vi "MegaAnalysis5.vi"() -> ()   [LabVIEW 2016] (continued)
                          n1538 = Multiply(x=w3837, y=6.283185307179586) -> (x*y=w3835:ext[])
                          n1539 = Divide(x=w3831, y=w3826) -> (x/y=w3839:ext[])
                          n1540 = Add(x=w3835, y=w3829) -> (x+y=w3832:ext[])
                          n1541 = Negate(x=w3839) -> (-x=w3838:ext[])
                          n1542 = Cosine(x=w3832) -> (cos(x)=w3833:ext[])
                          n1543 = Exponential(1:w3838) -> (0:w3834:ext[])
                          n1544 = Compound Arithmetic op=MULTIPLY(w3828, w3834, w3833) -> (w3825:ext[])
                          n1545 = call "writebinary.vi"(7:w3821, "base path"=w3823, "file index"=w3824, "data column"="dati", "data"=w3825) -> ()  [unwired: 7 out]
                        }
                        frame 2 {
                          w3843 = "dati"
                          n1546 = call "readbinary.vi"(7:w3840, "base path"=w3841, "file index"=w3842, "data column"="bcli") -> ("data"=w3846:ext[])  [unwired: 7 out]
                          n1547 = Divide(x=w3850, y=w3846) -> (x/y=w3858:ext[])
                          n1548 = Multiply(x=w3858, y=6.283185307179586) -> (x*y=w3856:ext[])
                          n1549 = call "readbinary.vi"(7:w3840, "base path"=w3841, "file index"=w3842, "data column"=w3843) -> ("data"=w3847:ext[])  [unwired: 7 out]
                          n1550 = Divide(x=w3851, y=w3846) -> (x/y=w3860:ext[])
                          n1551 = Add(x=w3856, y=w3849) -> (x+y=w3853:ext[])
                          n1552 = Negate(x=w3860) -> (-x=w3859:ext[])
                          n1553 = Cosine(x=w3853) -> (cos(x)=w3854:ext[])
                          n1554 = Exponential(1:w3859) -> (0:w3855:ext[])
                          n1555 = Compound Arithmetic op=MULTIPLY(w3848, w3855, w3854) -> (w3852:ext[])
                          n1556 = Subtract(x=w3847, y=w3852) -> (x-y=w3844:ext[])
                          n1557 = call "writebinary.vi"(7:w3840, "base path"=w3841, "file index"=w3842, "data column"=w3843, "data"=w3844) -> ()  [unwired: 7 out]
                        }
                        frame 3 {
                          w3864 = "dati"
                          n1558 = call "readbinary.vi"(7:w3861, "base path"=w3862, "file index"=w3863, "data column"="bcli") -> ("data"=w3866:ext[])  [unwired: 7 out]
                          n1559 = Reciprocal(x=w3866) -> (1/x=w3873:ext[])
                          n1560 = call "readbinary.vi"(7:w3861, "base path"=w3862, "file index"=w3863, "data column"=w3864) -> ("data"=w3867:ext[])  [unwired: 7 out]
                          n1561 = Index Array(array=w3873, index=2) -> (element=w3882:ext)
                          n1562 = Index Array(array=w3873, index=1) -> (element=w3883:ext)
                          n1563 = call <vilib>:"General Polynomial Fit.vi"("Y"=w3867, "polynomial order"="poly sub", "X"=w3873) -> ("Best Polynomial Fit"=w3871:dbl[])  [unwired: 9 in, 3 out]
                          n1564 = Subtract(x=w3883, y=w3882) -> (x-y=w3881:ext)
                          n1565 = Absolute Value(x=w3881) -> (abs(x)=w3880:ext)
                          n1566 = Reciprocal(x=w3880) -> (1/x=w3879:ext)
                          "sampling freq" <- w3879
                          n1567 = Subtract(x=w3867, y=w3871) -> (x-y=w3872:ext[])
                          n1568 = call-poly <vilib>:"Butterworth Filter.vi"("order"="order", "filter type"="filter type", "low cutoff freq: fl"="low cutoff", "high cutoff freq: fh"="high cutoff", "sampling freq: fs"=w3879, "X"=w3872) -> ("Filtered X"=w3869:dbl[])  [unwired: 1 in, 2 out]
                          n1569 = Add(x=w3869, y=w3871) -> (x+y=w3868:dbl[])
                          n1570 = case shown="False" "?" {
                            tunnel: w3869 -> [w3888 _]
                            tunnel: w3868 -> [_ w3895]
                            tunnel: w3864 -> [_ w3894]
                            tunnel: w3863 -> [w3889 w3893]
                            tunnel: w3862 -> [w3890 w3892]
                            tunnel: w3861 -> [w3886 w3891]
                            frame False {
                              n1571 = call "writebinary.vi"(7:w3886, "base path"=w3890, "file index"=w3889, "data column"="temp", "data"=w3888) -> ()  [unwired: 7 out]
                            }
                            frame True {
                              n1572 = call "writebinary.vi"(7:w3891, "base path"=w3892, "file index"=w3893, "data column"=w3894, "data"=w3895) -> ()  [unwired: 7 out]
                            }
                          }
                        }
                        frame 4 {
                          n1573 = call "readbinary.vi"(7:w3896, "base path"=w3898, "file index"=w3899, "data column"="timi") -> ("data"=w3903:ext[])  [unwired: 7 out]
                          n1574 = Multiply(x=w3903, y=6.283185307179586) -> (x*y=w3916:ext[])
                          n1575 = Multiply(x=w3916, y="f") -> (x*y=w3914:ext[])
                          n1576 = Add(x=w3914, y="phase") -> (x+y=w3912:ext[])
                          n1577 = call "readbinary.vi"(7:w3896, "base path"=w3898, "file index"=w3899, "data column"="bcli") -> ("data"=w3897:ext[])  [unwired: 7 out]
                          n1578 = Cosine(x=w3912) -> (cos(x)=w3911:ext[])
                          n1579 = Multiply(x=w3911, y="amp") -> (x*y=w3905:ext[])
                          n1580 = Divide(x="gamma", y=w3897) -> (x/y=w3908:ext[])
                          n1581 = Negate(x=w3908) -> (-x=w3907:ext[])
                          n1582 = Exponential(1:w3907) -> (0:w3906:ext[])
                          n1583 = Multiply(x=w3905, y=w3906) -> (x*y=w3901:ext[])
                          n1584 = call "writebinary.vi"(7:w3896, "base path"=w3898, "file index"=w3899, "data column"="dati", "data"=w3901) -> ()  [unwired: 7 out]
                        }
                      }
                    }
                  }
                  frame #5 {
                    n1585 = for {
                      tunnel: w3925 -> [_] mode=indexing
                      tunnel: "subtraction type" -> [w3935]
                      tunnel: "algorithm" -> [w3934]
                      tunnel: "polynomial order" -> [w3933]
                      tunnel: w3921 -> [w3928]
                      tunnel: "background subtraction method" -> [w3931]
                      tunnel: w3919 -> [w3927]
                      tunnel: [w3926] -> w3918 mode=indexing
                      i -> [w3929]
                      w3930 = "dati"
                      n1586 = call "readbinary.vi"(7:w3927, "base path"=w3928, "file index"=w3929, "data column"=w3930) -> ("data"=w3932:ext[])  [unwired: 7 out]
                      n1587 = case shown="2" w3935 {
                        tunnel: w3932 -> [w3952 w3962 w3973 w3980]
                        tunnel: [w3951 w3963 w3970 w3983] -> w3926
                        tunnel: w3934 -> [_ w3960 w3968 w3979]
                        tunnel: w3933 -> [_ w3959 w3969 w3978]
                        tunnel: w3929 -> [_ w3956 _ _]
                        tunnel: w3928 -> [_ w3955 _ _]
                        tunnel: w3927 -> [_ w3954 _ _]
                        frame 0, Default {
                          n1588 = Multiply(x=w3952, y=0) -> (x*y=w3951:ext[])
                        }
                        frame 1 {
                          n1589 = call "readbinary.vi"(7:w3954, "base path"=w3955, "file index"=w3956, "data column"="temp") -> ("data"=w3958:ext[])  [unwired: 7 out]
                          n1590 = Subtract(x=w3962, y=w3958) -> (x-y=w3961:ext[])
                          n1591 = Array Size(array=w3962) -> (size(s)=w3965:i32)
                          n1592 = for {
                            N: w3965 -> [_]
                            tunnel: [w3967] -> w3966 mode=indexing
                            i -> [w3967]
                          }
                          n1593 = Divide(x=w3966, y=w3965) -> (x/y=w3964:dbl[])
                          n1594 = call <vilib>:"General Polynomial Fit.vi"("Y"=w3961, "polynomial order"=w3959, "X"=w3964, "algorithm"=w3960) -> ("Best Polynomial Fit"=w3963:dbl[])  [unwired: 8 in, 3 out]
                        }
                        frame 2 {
                          n1595 = Natural Logarithm(1:w3973) -> (0:w3971:ext[])
                          n1596 = Array Size(array=w3973) -> (size(s)=w3975:i32)
                          n1597 = for {
                            N: w3975 -> [_]
                            tunnel: [w3977] -> w3976 mode=indexing
                            i -> [w3977]
                          }
                          n1598 = Divide(x=w3976, y=w3975) -> (x/y=w3974:dbl[])
                          n1599 = call <vilib>:"General Polynomial Fit.vi"("Y"=w3971, "polynomial order"=w3969, "X"=w3974, "algorithm"=w3968) -> ("Best Polynomial Fit"=w3972:dbl[])  [unwired: 8 in, 3 out]
                          n1600 = Exponential (Arg) -1(1:w3972) -> (0:w3970:dbl[])
                        }
                        frame 3 {
                          n1601 = Reciprocal(x=w3980) -> (1/x=w3981:ext[])
                          n1602 = Array Size(array=w3980) -> (size(s)=w3985:i32)
                          n1603 = for {
                            N: w3985 -> [_]
                            tunnel: [w3987] -> w3986 mode=indexing
                            i -> [w3987]
                          }
                          n1604 = Divide(x=w3986, y=w3985) -> (x/y=w3984:dbl[])
                          n1605 = call <vilib>:"General Polynomial Fit.vi"("Y"=w3981, "polynomial order"=w3978, "X"=w3984, "algorithm"=w3979) -> ("Best Polynomial Fit"=w3982:dbl[])  [unwired: 8 in, 3 out]
                          n1606 = Reciprocal(x=w3982) -> (1/x=w3983:dbl[])
                        }
                      }
                      n1607 = case shown="2" w3931 {
                        tunnel: w3932 -> [_ w3942 w3950]
                        tunnel: w3926 -> [_ w3941 w3948]
                        tunnel: w3930 -> [_ w3939 w3946]
                        tunnel: w3929 -> [_ w3938 w3945]
                        tunnel: w3928 -> [_ w3937 w3944]
                        tunnel: w3927 -> [_ w3936 w3943]
                        frame 0, Default {
                        }
                        frame 1 {
                          n1608 = Subtract(x=w3942, y=w3941) -> (x-y=w3940:ext[])
                          n1609 = call "writebinary.vi"(7:w3936, "base path"=w3937, "file index"=w3938, "data column"=w3939, "data"=w3940) -> ()  [unwired: 7 out]
                        }
                        frame 2 {
                          n1610 = Divide(x=w3950, y=w3948) -> (x/y=w3949:ext[])
                          n1611 = Decrement(x=w3949) -> (x-1=w3947:ext[])
                          n1612 = call "writebinary.vi"(7:w3943, "base path"=w3944, "file index"=w3945, "data column"=w3946, "data"=w3947) -> ()  [unwired: 7 out]
                        }
                      }
                    }
                  }
                  frame #6 {
                    n1613 = for {
                      tunnel: "post interp amplitude/field modifier" -> [w3997]
                      tunnel: w3991 -> [_] mode=indexing
                      tunnel: w3990 -> [w3995]
                      tunnel: w3989 -> [w3994]
                      tunnel: w3988 -> [w3993] mode=indexing
                      i -> [w3996]
                      n1614 = case shown="4" w3997 {
                        tunnel: w3996 -> [_ w4001 w4013 w4029 w4053 w4060]
                        tunnel: w3995 -> [_ w4000 w4012 w4028 w4052 w4059]
                        tunnel: w3994 -> [_ w3998 w4009 w4027 w4051 w4058]
                        tunnel: w3993 -> [_ _ _ _ _ w4057]
                        frame 0, Default {
                        }
                        frame 1 {
                          w4003 = "dati"
                          n1615 = call "readbinary.vi"(7:w3998, "base path"=w4000, "file index"=w4001, "data column"=w4003) -> ("data"=w4005:ext[])  [unwired: 7 out]
                          n1616 = call "readbinary.vi"(7:w3998, "base path"=w4000, "file index"=w4001, "data column"="bcli") -> ("data"=w4002:ext[])  [unwired: 7 out]
                          n1617 = Divide(x="gamma", y=w4002) -> (x/y=w4007:ext[])
                          n1618 = Exponential(1:w4007) -> (0:w4006:ext[])
                          n1619 = Multiply(x=w4005, y=w4006) -> (x*y=w4004:ext[])
                          n1620 = call "writebinary.vi"(7:w3998, "base path"=w4000, "file index"=w4001, "data column"=w4003, "data"=w4004) -> ()  [unwired: 7 out]
                        }
                        frame 2 {
                          w4014 = "dati"
                          n1621 = call "readbinary.vi"(7:w4009, "base path"=w4012, "file index"=w4013, "data column"=w4014) -> ("data"=w4016:ext[])  [unwired: 7 out]
                          n1622 = call "readbinary.vi"(7:w4009, "base path"=w4012, "file index"=w4013, "data column"="bcli") -> ("data"=w4011:ext[])  [unwired: 7 out]
                          n1623 = for {
                            shift-right: [w4024] -> _
                            shift-left: 0 -> [w4026]
                            tunnel: w4016 -> [w4024] mode=indexing
                            tunnel: [w4025] -> w4019 mode=indexing
                            n1624 = Subtract(x=w4024, y=w4026) -> (x-y=w4025:ext)
                          }
                          n1625 = Index Array(array=w4011, index=1) -> (element=w4021:ext)
                          n1626 = Index Array(array=w4011, index=0) -> (element=w4020:ext)
                          n1627 = Subtract(x=w4021, y=w4020) -> (x-y=w4018:ext)
                          n1628 = Divide(x=w4019, y=w4018) -> (x/y=w4015:ext[])
                          n1629 = call "writebinary.vi"(7:w4009, "base path"=w4012, "file index"=w4013, "data column"=w4014, "data"=w4015) -> ()  [unwired: 7 out]
                        }
                        frame 3 {
                          w4030 = "dati"
                          n1630 = call "readbinary.vi"(7:w4027, "base path"=w4028, "file index"=w4029, "data column"="bcli") -> ("data"=w4034:ext[])  [unwired: 7 out]
                          n1631 = call "readbinary.vi"(7:w4027, "base path"=w4028, "file index"=w4029, "data column"=w4030) -> ("data"=w4032:ext[])  [unwired: 7 out]
                          n1632 = for {
                            shift-right: [w4048] -> _
                            shift-left: 0 -> [w4050]
                            tunnel: w4032 -> [w4048] mode=indexing
                            tunnel: [w4049] -> w4040 mode=indexing
                            n1633 = Subtract(x=w4048, y=w4050) -> (x-y=w4049:ext)
                          }
                          n1634 = Index Array(array=w4034, index=1) -> (element=w4042:ext)
                          n1635 = Index Array(array=w4034, index=0) -> (element=w4041:ext)
                          n1636 = Subtract(x=w4042, y=w4041) -> (x-y=w4036:ext)
                          n1637 = Divide(x=w4040, y=w4036) -> (x/y=w4035:ext[])
                          n1638 = for {
                            shift-right: [w4045] -> _
                            shift-left: 0 -> [w4047]
                            tunnel: w4035 -> [w4045] mode=indexing
                            tunnel: [w4046] -> w4038 mode=indexing
                            n1639 = Subtract(x=w4045, y=w4047) -> (x-y=w4046:ext)
                          }
                          n1640 = Divide(x=w4038, y=w4036) -> (x/y=w4031:ext[])
                          n1641 = call "writebinary.vi"(7:w4027, "base path"=w4028, "file index"=w4029, "data column"=w4030, "data"=w4031) -> ()  [unwired: 7 out]
                        }
                        frame 4 {
                          w4054 = "dati"
                          n1642 = call "readbinary.vi"(7:w4051, "base path"=w4052, "file index"=w4053, "data column"=w4054) -> ("data"=w4056:ext[])  [unwired: 7 out]
                          n1643 = call-poly <vilib>:"Hanning Window.vi"("X"=w4056) -> ("Windowed X"=w4055:dbl[])  [unwired: 1 out]
                          n1644 = call "writebinary.vi"(7:w4051, "base path"=w4052, "file index"=w4053, "data column"=w4054, "data"=w4055) -> ()  [unwired: 7 out]
                        }
                        frame 5 {
                          w4061 = "dati"
                          n1645 = call "readbinary.vi"(7:w4058, "base path"=w4059, "file index"=w4060, "data column"=w4061) -> ()  [unwired: 8 out]
                          n1646 = call "writebinary.vi"(7:w4058, "base path"=w4059, "file index"=w4060, "data column"=w4061, "data"=w4057) -> ()  [unwired: 7 out]
                        }
                      }
                    }
                  }
                  frame #7 {
                  }
                }
                n1647 = global write "status.vi" "String"("interpolating") -> ()
              }
            }
          }
          frame #2 {
            n1648 = Equal?(x=3, y=w4074) -> (x = y?=w4066:bool)
            n1649 = Equal?(x=w4072, y=2) -> (x = y?=w4065:bool)
            n1650 = And(x=w4066, y=w4065) -> (x .and. y?=w4064:bool)
            n1651 = stacked-sequence {
              seq-local: [w4077 _ _] -> [_ w4195 _]
              seq-local: [w4076 _ _] -> [_ w4193 w4209]
              tunnel: w4070 -> [w4088 _ w4204]
              tunnel: w4069 -> [w4081 _ w4208]
              tunnel: w4068 -> [w4079 _ w4207]
              tunnel: "cut off selection" -> [w4078 _ _]
              tunnel: w4064 -> [_ w4196 _]
              tunnel: w4063 -> [_ _ w4203]
              tunnel: w4062 -> [w4075 _ w4202]
              frame #0 {
                n1652 = Build Path(base path=w4081, name or relative path="files3") -> (appended path=w4086:path)
                n1653 = call-poly <vilib>:"Read From Spreadsheet File.vi"("file path (dialog if empty)"=w4086) -> ("first row"=w4085:string[])  [unwired: 3 in, 7 out]
                n1654 = call "readbinary.vi"("base path"=w4081, "file index"=0, "data column"="inte") -> ("data"=w4083:ext[])  [unwired: 1 in, 7 out]
                n1655 = Index Array(array=w4083) -> (element=w4080:ext)  [unwired: 1 in]
                "interpolate in:" <- w4080
                n1656 = case shown="True" w4088 {
                  tunnel: w4085 -> [_ w4099]
                  tunnel: w4081 -> [_ w4098]
                  tunnel: w4080 -> [_ w4097]
                  tunnel: w4079 -> [_ w4096]
                  tunnel: w4078 -> [_ w4095]
                  tunnel: [w4089 w4094] -> w4077
                  tunnel: [w4089 w4093] -> w4076
                  tunnel: w4075 -> [_ w4092]
                  frame False {
                    w4091 = dbl[] [] ("Array 13")
                    n1657 = Bundle("Array 13"=w4091, "Array 13"=w4091) -> (w4090:cluster{"Array 13":dbl[], "Array 13":dbl[]})  [unwired: 1 out]
                    n1658 = Build Array(w4090) -> (w4089:cluster{"Array 13":dbl[], "Array 13":dbl[]}[])
                  }
                  frame True {
                    n1659 = for {
                      tunnel: w4099 -> [_] mode=indexing
                      tunnel: w4098 -> [w4127]
                      tunnel: w4097 -> [w4130]
                      tunnel: w4096 -> [w4129]
                      tunnel: w4095 -> [w4117]
                      tunnel: [w4110] -> w4094 mode=indexing
                      tunnel: [w4105] -> w4093 mode=indexing
                      tunnel: w4092 -> [w4100]
                      i -> [w4128]
                      n1660 = case shown="2" w4130 {
                        tunnel: w4128 -> [w4174 w4179 w4185 w4190]
                        tunnel: w4127 -> [w4173 w4178 w4184 w4189]
                        tunnel: [w4172 w4177 w4182 w4188] -> w4106
                        tunnel: w4100 -> [w4171 w4176 w4181 w4187]
                        frame 0, Default {
                          n1661 = call "readbinary.vi"(7:w4171, "base path"=w4173, "file index"=w4174, "data column"="timi") -> ("data"=w4172:ext[])  [unwired: 7 out]
                        }
                        frame 1 {
                          n1662 = call "readbinary.vi"(7:w4176, "base path"=w4178, "file index"=w4179, "data column"="bcli") -> ("data"=w4177:ext[])  [unwired: 7 out]
                        }
                        frame 2 {
                          n1663 = call "readbinary.vi"(7:w4181, "base path"=w4184, "file index"=w4185, "data column"="bcli") -> ("data"=w4183:ext[])  [unwired: 7 out]
                          n1664 = Reciprocal(x=w4183) -> (1/x=w4182:ext[])
                        }
                        frame 3 {
                          n1665 = call "readbinary.vi"(7:w4187, "base path"=w4189, "file index"=w4190, "data column"="dati") -> ("data"=w4188:ext[])  [unwired: 7 out]
                        }
                      }
                      n1666 = case shown="0, Default" w4129 {
                        tunnel: w4128 -> [w4153 w4158 w4164 w4169]
                        tunnel: w4127 -> [w4152 w4157 w4163 w4168]
                        tunnel: [w4151 w4156 w4161 w4167] -> w4126
                        tunnel: w4100 -> [w4150 w4155 w4160 w4166]
                        frame 0, Default {
                          n1667 = call "readbinary.vi"(7:w4150, "base path"=w4152, "file index"=w4153, "data column"="timi") -> ("data"=w4151:ext[])  [unwired: 7 out]
                        }
                        frame 1 {
                          n1668 = call "readbinary.vi"(7:w4155, "base path"=w4157, "file index"=w4158, "data column"="bcli") -> ("data"=w4156:ext[])  [unwired: 7 out]
                        }
                        frame 2 {
                          n1669 = call "readbinary.vi"(7:w4160, "base path"=w4163, "file index"=w4164, "data column"="bcli") -> ("data"=w4162:ext[])  [unwired: 7 out]
                          n1670 = Reciprocal(x=w4162) -> (1/x=w4161:ext[])
                        }
                        frame 3 {
                          n1671 = call "readbinary.vi"(7:w4166, "base path"=w4168, "file index"=w4169, "data column"="dati") -> ("data"=w4167:ext[])  [unwired: 7 out]
                        }
                      }
                      n1672 = Array Size(array=w4106) -> (size(s)=w4116:i32)
                      n1673 = Index Array(array=w4106, index=0) -> (element=w4120:ext)
                      n1674 = call-poly <vilib>:"Scaled Time Domain Window.vi"("window"="window", "X"=w4126) -> ("Windowed X"=w4125:dbl[])  [unwired: 1 in, 8 out]
                      n1675 = Decrement(x=w4116) -> (x-1=w4123:i32)
                      n1676 = Index Array(array=w4106, index=w4123) -> (element=w4121:ext)
                      n1677 = Subtract(x=w4121, y=w4120) -> (x-y=w4119:ext)
                      n1678 = call-poly <vilib>:"FFT.vi"("X"=w4125) -> ("FFT {X}"=w4124:cdb[])  [unwired: 2 in, 8 out]
                      n1679 = Absolute Value(x=w4119) -> (abs(x)=w4118:ext)
                      n1680 = Complex To Polar(r * e^(i*theta)=w4124) -> (r=w4109:dbl[], theta=w4108:dbl[])
                      n1681 = Reciprocal(x=w4118) -> (1/x=w4112:ext)
                      n1682 = for {
                        shift-right: [w4140] -> w4107
                        shift-left: w4109 -> [w4138]
                        tunnel: w4117 -> [w4148] mode=indexing
                        tunnel: w4112 -> [w4139]
                        n1683 = Unbundle(w4148) -> ("lower limit"=w4147:dbl, "upper limit"=w4146:dbl, "cuttoff multiplier"=w4134:dbl)
                        n1684 = Divide(x=w4147, y=w4139) -> (x/y=w4136:ext)
                        n1685 = Divide(x=w4146, y=w4139) -> (x/y=w4145:ext)
                        n1686 = Subtract(x=w4145, y=w4136) -> (x-y=w4144:ext)
                        n1687 = Increment(x=w4144) -> (x+1=w4137:ext)
                        n1688 = Array Subset(array=w4138, index=w4136, length=w4137) -> (w4135:dbl[])
                        n1689 = Multiply(x=w4135, y=w4134) -> (x*y=w4133:dbl[])
                        n1690 = Replace Array Subset(array=w4138, new element=w4133, index=w4136) -> (w4143:dbl[])
                        n1691 = Reverse 1D Array(array=w4143) -> (reversed array=w4142:dbl[])
                        n1692 = for {
                          N: w4137 -> [_]
                          tunnel: [0] -> _ mode=indexing
                        }
                        n1693 = Replace Array Subset(array=w4142, new element=w4133, index=w4136) -> (w4141:dbl[])
                        n1694 = Reverse 1D Array(array=w4141) -> (reversed array=w4140:dbl[])
                      }
                      n1695 = for {
                        N: w4116 -> [_]
                        tunnel: [1] -> w4114 mode=indexing
                        tunnel: [w4131] -> w4113 mode=indexing
                        i -> [w4131]
                      }
                      n1696 = call-poly <vilib>:"Scaled Time Domain Window.vi"("window"="window", "X"=w4114) -> ("Windowed X"=w4102:dbl[])  [unwired: 1 in, 8 out]
                      n1697 = Multiply(x=w4113, y=w4112) -> (x*y=w4111:ext[])
                      n1698 = Polar To Complex(1:w4108, 2:w4107) -> (0:w4101:cdb[])
                      n1699 = call-poly <vilib>:"Inverse FFT.vi"("FFT {X}"=w4101) -> ("X"=w4104:dbl[])  [unwired: 1 in, 9 out]
                      n1700 = Divide(x=w4104, y=w4102) -> (x/y=w4103:dbl[])
                      n1701 = Bundle(w4111, w4107) -> (w4110:cluster{ext[], dbl[]})  [unwired: 1 out]
                      n1702 = Bundle("data"=w4106, w4103) -> (w4105:cluster{"data":ext[], dbl[]})  [unwired: 1 out]
                    }
                  }
                }
              }
              frame #1 {
                n1703 = case shown="False" w4196 {
                  tunnel: w4195 -> [_ w4201]
                  tunnel: [w4197 w4201] -> w4194
                  tunnel: w4193 -> [_ w4200]
                  tunnel: [w4197 w4200] -> w4192
                  frame False {
                    w4199 = dbl[] [] ("Array 14")
                    n1704 = Bundle("Array 14"=w4199, "Array 14"=w4199) -> (w4198:cluster{"Array 14":dbl[], "Array 14":dbl[]})  [unwired: 1 out]
                    n1705 = Build Array(w4198) -> (w4197:cluster{"Array 14":dbl[], "Array 14":dbl[]}[])
                  }
                  frame True {
                  }
                }
                "?" <- w4194
                "?" <- w4192
              }
              frame #2 {
                n1706 = And(x=w4203, y=w4204) -> (x .and. y?=w4205:bool)
                n1707 = stacked-sequence {
                  tunnel: w4209 -> [w4214 w4247 w4280]
                  tunnel: w4208 -> [w4213 w4246 w4279]
                  tunnel: w4207 -> [w4212 w4245 w4278]
                  tunnel: "?" -> [_ _ w4277]
                  tunnel: w4205 -> [w4211 w4244 _]
                  tunnel: w4202 -> [w4210 w4243 w4276]
                  frame #0 {
                    n1708 = case shown="False" w4211 {
                      tunnel: w4214 -> [_ w4218]
                      tunnel: w4213 -> [_ w4217]
                      tunnel: w4212 -> [_ w4216]
                      tunnel: w4210 -> [_ w4215]
                      frame False {
                      }
                      frame True {
                        n1709 = for {
                          tunnel: w4218 -> [_] mode=indexing
                          tunnel: w4217 -> [w4220]
                          tunnel: w4216 -> [w4224]
                          tunnel: w4215 -> [w4219]
                          i -> [w4221]
                          n1710 = case shown="0, Default" w4224 {
                            tunnel: w4221 -> [w4227 w4231 w4236 w4241]
                            tunnel: w4220 -> [w4226 w4230 w4235 w4240]
                            tunnel: [w4225 w4229 w4233 w4239] -> w4223
                            tunnel: w4219 -> [_ _ _ w4238]
                            frame 0, Default {
                              n1711 = call "readbinary.vi"("base path"=w4226, "file index"=w4227, "data column"="timi") -> ("data"=w4225:ext[])  [unwired: 1 in, 7 out]
                            }
                            frame 1 {
                              n1712 = call "readbinary.vi"("base path"=w4230, "file index"=w4231, "data column"="bcli") -> ("data"=w4229:ext[])  [unwired: 1 in, 7 out]
                            }
                            frame 2 {
                              n1713 = call "readbinary.vi"("base path"=w4235, "file index"=w4236, "data column"="bcli") -> ("data"=w4234:ext[])  [unwired: 1 in, 7 out]
                              n1714 = Reciprocal(x=w4234) -> (1/x=w4233:ext[])
                            }
                            frame 3 {
                              n1715 = call "readbinary.vi"(7:w4238, "base path"=w4240, "file index"=w4241, "data column"="dati") -> ("data"=w4239:ext[])  [unwired: 7 out]
                            }
                          }
                          n1716 = call "writebinary.vi"(7:w4219, "base path"=w4220, "file index"=w4221, "data column"="hold", "data"=w4223) -> ()  [unwired: 7 out]
                        }
                      }
                    }
                  }
                  frame #1 {
                    n1717 = case shown="True" w4244 {
                      tunnel: w4247 -> [_ w4251]
                      tunnel: w4246 -> [_ w4250]
                      tunnel: w4245 -> [_ w4249]
                      tunnel: w4243 -> [_ w4248]
                      frame False {
                      }
                      frame True {
                        n1718 = for {
                          tunnel: w4251 -> [w4257] mode=indexing
                          tunnel: w4250 -> [w4256]
                          tunnel: w4249 -> [w4253]
                          tunnel: w4248 -> [w4252]
                          i -> [w4255]
                          n1719 = Unbundle(w4257) -> ("Array 13"=w4254:dbl[])  [unwired: 1 out]
                          n1720 = case shown="0, Default" w4253 {
                            tunnel: w4255 -> [w4260 w4264 w4269 w4274]
                            tunnel: w4256 -> [w4261 w4265 w4270 w4275]
                            tunnel: w4254 -> [w4258 w4262 w4267 w4272]
                            tunnel: w4252 -> [_ _ _ w4271]
                            frame 0, Default {
                              n1721 = call "writebinary.vi"("base path"=w4261, "file index"=w4260, "data column"="timi", "data"=w4258) -> ()  [unwired: 1 in, 7 out]
                            }
                            frame 1 {
                              n1722 = call "writebinary.vi"("base path"=w4265, "file index"=w4264, "data column"="bcli", "data"=w4262) -> ()  [unwired: 1 in, 7 out]
                            }
                            frame 2 {
                              n1723 = Reciprocal(x=w4267) -> (1/x=w4266:dbl[])
                              n1724 = call "writebinary.vi"("base path"=w4270, "file index"=w4269, "data column"="bcli", "data"=w4266) -> ()  [unwired: 1 in, 7 out]
                            }
                            frame 3 {
                              n1725 = call "writebinary.vi"(7:w4271, "base path"=w4275, "file index"=w4274, "data column"="dati", "data"=w4272) -> ()  [unwired: 7 out]
                            }
                          }
                        }
                      }
                    }
                  }
                  frame #2 {
                    n1726 = case shown="True" w4277 {
                      tunnel: w4280 -> [_ w4284]
                      tunnel: w4279 -> [_ w4283]
                      tunnel: w4278 -> [_ w4282]
                      tunnel: w4276 -> [_ w4281]
                      frame False {
                      }
                      frame True {
                        n1727 = for {
                          tunnel: w4284 -> [_] mode=indexing
                          tunnel: w4283 -> [w4287]
                          tunnel: w4282 -> [w4290]
                          tunnel: w4281 -> [w4285]
                          i -> [w4288]
                          n1728 = call "readbinary.vi"(7:w4285, "base path"=w4287, "file index"=w4288, "data column"="hold") -> ("data"=w4286:ext[])  [unwired: 7 out]
                          n1729 = case shown="2" w4290 {
                            tunnel: w4288 -> [w4294 w4299 w4305 w4310]
                            tunnel: w4287 -> [w4295 w4300 w4306 w4311]
                            tunnel: w4286 -> [w4292 w4297 w4302 w4308]
                            tunnel: w4285 -> [w4291 w4296 w4301 w4307]
                            frame 0, Default {
                              n1730 = call "writebinary.vi"(7:w4291, "base path"=w4295, "file index"=w4294, "data column"="timi", "data"=w4292) -> ()  [unwired: 7 out]
                            }
                            frame 1 {
                              n1731 = call "writebinary.vi"(7:w4296, "base path"=w4300, "file index"=w4299, "data column"="bcli", "data"=w4297) -> ()  [unwired: 7 out]
                            }
                            frame 2 {
                              n1732 = Reciprocal(x=w4302) -> (1/x=w4303:ext[])
                              n1733 = call "writebinary.vi"(7:w4301, "base path"=w4306, "file index"=w4305, "data column"="bcli", "data"=w4303) -> ()  [unwired: 7 out]
                            }
                            frame 3 {
                              n1734 = call "writebinary.vi"(7:w4307, "base path"=w4311, "file index"=w4310, "data column"="dati", "data"=w4308) -> ()  [unwired: 7 out]
                            }
                          }
                        }
                      }
                    }
                  }
                }
              }
            }
          }
          frame #3 {
            w4314 = 0
            n1735 = And(x=w4323, y="?") -> (x .and. y?=w4324:bool)
            n1736 = Build Path(base path=w4316, name or relative path="files3") -> (appended path=w4320:path)
            n1737 = call-poly <vilib>:"Read From Spreadsheet File.vi"("file path (dialog if empty)"=w4320) -> ("first row"=w4317:string[])  [unwired: 3 in, 7 out]
            n1738 = call "readbinary.vi"("base path"=w4316, "file index"=w4314, "data column"="inte") -> ("data"=w4319:ext[])  [unwired: 1 in, 7 out]
            n1739 = Index Array(array=w4319, index=w4314) -> (element=w4315:ext)
            n1740 = case shown="True" w4324 {
              tunnel: w4317 -> [_ w4329]
              tunnel: w4316 -> [_ w4328]
              tunnel: w4315 -> [_ w4327]
              tunnel: w4313 -> [_ w4326]
              tunnel: w4312 -> [_ w4325]
              frame False {
              }
              frame True {
                n1741 = for {
                  tunnel: w4329 -> [_] mode=indexing
                  tunnel: w4328 -> [w4332]
                  tunnel: w4327 -> [_]
                  tunnel: w4326 -> [w4334]
                  tunnel: w4325 -> [w4330]
                  i -> [w4333]
                  n1742 = case shown="3" w4334 {
                    tunnel: w4333 -> [w4356 w4362 w4367 w4373 w4378]
                    tunnel: w4332 -> [w4355 w4361 w4366 w4372 w4377]
                    tunnel: [w4354 w4360 w4365 w4369 w4376] -> w4331
                    tunnel: w4330 -> [w4353 w4358 w4363 w4368 w4374]
                    frame 0, Default {
                      n1743 = call "readbinary.vi"(7:w4353, "base path"=w4355, "file index"=w4356, "data column"="timi") -> ("data"=w4354:ext[])  [unwired: 7 out]
                    }
                    frame 1 {
                      n1744 = call "readbinary.vi"(7:w4358, "base path"=w4361, "file index"=w4362, "data column"="bdti") -> ("data"=w4360:ext[])  [unwired: 7 out]
                    }
                    frame 2 {
                      n1745 = call "readbinary.vi"(7:w4363, "base path"=w4366, "file index"=w4367, "data column"="bcli") -> ("data"=w4365:ext[])  [unwired: 7 out]
                    }
                    frame 3 {
                      n1746 = call "readbinary.vi"(7:w4368, "base path"=w4372, "file index"=w4373, "data column"="bcli") -> ("data"=w4370:ext[])  [unwired: 7 out]
                      n1747 = Reciprocal(x=w4370) -> (1/x=w4369:ext[])
                    }
                    frame 4 {
                      n1748 = call "readbinary.vi"(7:w4374, "base path"=w4377, "file index"=w4378, "data column"="dati") -> ("data"=w4376:ext[])  [unwired: 7 out]
                    }
                  }
                  n1749 = Subtract(x=w4331, y="lower") -> (x-y=w4349:ext[])
                  n1750 = Subtract(x=w4331, y="upper") -> (x-y=w4350:ext[])
                  n1751 = Absolute Value(x=w4349) -> (abs(x)=w4347:ext[])
                  n1752 = Absolute Value(x=w4350) -> (abs(x)=w4348:ext[])
                  n1753 = Array Max & Min(array=w4347) -> (min index (indices)=w4343:i32)  [unwired: 3 out]
                  n1754 = Array Max & Min(array=w4348) -> (min index (indices)=w4335:i32)  [unwired: 3 out]
                  n1755 = Build Array("timi", "bdti", "bcli", "dati") -> (w4338:string[])
                  n1756 = Less?(x=w4335, y=w4343) -> (x < y?=w4344:bool)
                  n1757 = Subtract(x=w4335, y=w4343) -> (x-y=w4346:i32)
                  n1758 = Absolute Value(x=w4346) -> (abs(x)=w4345:i32)
                  n1759 = Select(t=w4335, s=w4344, f=w4343) -> (s? t:f=w4337:i32)
                  n1760 = Increment(x=w4345) -> (x+1=w4336:i32)
                  n1761 = for {
                    tunnel: w4338 -> [w4382] mode=indexing
                    tunnel: w4333 -> [w4381]
                    tunnel: w4332 -> [w4380]
                    tunnel: w4337 -> [w4385]
                    tunnel: w4336 -> [w4384]
                    tunnel: w4330 -> [w4379]
                    n1762 = call "readbinary.vi"(7:w4379, "base path"=w4380, "file index"=w4381, "data column"=w4382) -> ("data"=w4386:ext[])  [unwired: 7 out]
                    n1763 = Array Subset(array=w4386, index=w4385, length=w4384) -> (w4383:ext[])
                    n1764 = call "writebinary.vi"(7:w4379, "base path"=w4380, "file index"=w4381, "data column"=w4382, "data"=w4383) -> ()  [unwired: 7 out]
                  }
                }
              }
            }
          }
          frame #4 {
            n1765 = Build Array("timi", "bdti", "bcli", "dati") -> (w4389:string[])
            n1766 = case shown="True" "?" {
              tunnel: w4395 -> [_ w4399]
              tunnel: w4389 -> [_ w4398]
              tunnel: w4388 -> [_ w4397]
              tunnel: w4387 -> [_ w4396]
              frame False {
              }
              frame True {
                n1767 = case shown="True" w4397 {
                  tunnel: w4399 -> [_ w4402]
                  tunnel: w4398 -> [_ w4401]
                  tunnel: w4396 -> [_ w4400]
                  frame False {
                  }
                  frame True {
                    n1768 = stacked-sequence {
                      seq-local: [w4413 _] -> [_ w4444]
                      seq-local: [w4414 _] -> [_ w4447]
                      seq-local: [w4405 _] -> [_ w4438]
                      seq-local: [w4404 _] -> [_ w4436]
                      tunnel: w4402 -> [w4409 _]
                      tunnel: w4401 -> [w4412 _]
                      tunnel: w4400 -> [w4403 _]
                      frame #0 {
                        n1769 = Build Path(base path=w4409, name or relative path="paths3") -> (appended path=w4404:path)
                        n1770 = Build Path(base path=w4409, name or relative path="files3") -> (appended path=w4405:path)
                        n1771 = call "readbinary.vi"(7:w4403, "base path"=w4409, "file index"=0, "data column"="dati") -> ("data"=w4408:ext[])  [unwired: 7 out]
                        n1772 = call-poly <vilib>:"Read From Spreadsheet File.vi"("file path (dialog if empty)"=w4404) -> ("first row"=w4415:string[])  [unwired: 3 in, 7 out]
                        n1773 = Array Size(array=w4408) -> (size(s)=w4407:i32)
                        n1774 = for {
                          N: w4407 -> [_]
                          tunnel: [0] -> w4406 mode=indexing
                        }
                        n1775 = call-poly <vilib>:"Read From Spreadsheet File.vi"("file path (dialog if empty)"=w4405) -> ("first row"=w4413:string[])  [unwired: 3 in, 7 out]
                        n1776 = String To Path(string=w4415) -> (path=w4414:path[])
                        n1777 = for {
                          tunnel: w4413 -> [w4426]
                          tunnel: w4412 -> [w4423] mode=indexing
                          tunnel: w4409 -> [w4422]
                          tunnel: w4406 -> [w4427]
                          tunnel: w4403 -> [w4419]
                          n1778 = Array Size(array=w4426) -> (size(s)=w4421:i32)
                          n1779 = for {
                            N: w4421 -> [_]
                            tunnel: w4426 -> [_] mode=indexing
                            tunnel: w4422 -> [w4434]
                            shift-right: [w4433] -> w4425
                            shift-left: w4427 -> [w4431]
                            tunnel: w4423 -> [w4430]
                            tunnel: w4419 -> [w4428]
                            i -> [w4429]
                            n1780 = call "readbinary.vi"(7:w4428, "base path"=w4434, "file index"=w4429, "data column"=w4430) -> ("data"=w4432:ext[])  [unwired: 7 out]
                            n1781 = Add(x=w4432, y=w4431) -> (x+y=w4433:ext[])
                          }
                          n1782 = Divide(x=w4425, y=w4421) -> (x/y=w4424:ext[])
                          n1783 = call "writebinary.vi"(7:w4419, "base path"=w4422, "file index"=0, "data column"=w4423, "data"=w4424) -> ()  [unwired: 7 out]
                        }
                      }
                      frame #1 {
                        n1784 = Index Array(array=w4447, index=0) -> (element=w4441:path)
                        n1785 = case shown="True" "?" {
                          tunnel: w4444 -> [w4451 w4455]
                          tunnel: "append string onto file name" -> [w4450 w4456]
                          tunnel: "?" -> [_ w4454]
                          tunnel: [w4448 w4453] -> w4440
                          frame False {
                            n1786 = Index Array(array=w4451, index=0) -> (element=w4449:string)
                            n1787 = Concatenate Strings(w4450, w4449) -> (w4448:string)
                          }
                          frame True {
                            n1788 = for {
                              shift-right: [w4457] -> w4453
                              shift-left: w4456 -> [w4459]
                              tunnel: w4455 -> [w4462] mode=indexing
                              tunnel: w4454 -> [w4460]
                              n1789 = String Subset(string=w4462, offset (0)=0, length (rest)=w4460) -> (substring=w4458:string)
                              n1790 = Concatenate Strings(w4459, w4458) -> (w4457:string)
                            }
                          }
                        }
                        n1791 = Build Array(w4441) -> (w4439:path[])
                        n1792 = Path To String(path=w4439) -> (string=w4435:string[])
                        n1793 = Build Array(w4440) -> (w4437:string[])
                        n1794 = call-poly <vilib>:"Write To Spreadsheet File.vi"("1D data"=w4437, "file path (dialog if empty)"=w4438) -> ()  [unwired: 4 in, 3 out]
                        n1795 = call-poly <vilib>:"Write To Spreadsheet File.vi"("1D data"=w4435, "file path (dialog if empty)"=w4436) -> ()  [unwired: 4 in, 3 out]
                      }
                    }
                  }
                }
              }
            }
          }
          frame #5 {
            w4466 = FALSE  # Set axes names
            n1796 = Equal?(x=3, y=w4472) -> (x = y?=w4477:bool)
            n1797 = Build Path(base path=w4480, name or relative path="files3") -> (appended path=w4478:path)
            n1798 = Equal?(x=w4473, y=4) -> (x = y?=w4476:bool)
            n1799 = And(x=w4477, y=w4476) -> (x .and. y?=w4471:bool)
            n1800 = call-poly <vilib>:"Read From Spreadsheet File.vi"("file path (dialog if empty)"=w4478) -> ("first row"=w4467:string[])  [unwired: 3 in, 7 out]
            "files" <- w4467
            n1801 = case shown="1" "label" {
              tunnel: w4467 -> [w4482 _ _]
              tunnel: [w4482 w4485 w4490] -> w4464
              frame 0, Default {
              }
              frame 1 {
                n1802 = property on="angle theta (cos theta renorm.)" class="Arr (strict)"() -> ("Value"=w4486:ext[])  [unwired: 2 in, 2 out]
                n1803 = Number To Fractional String(number=w4486, width (-)=10, precision (6)=3) -> (F-format string=w4485:string[])  [unwired: 1 out]
              }
              frame 2 {
                n1804 = property on="variable (T)" class="Arr (strict)"() -> ("Value"=w4489:dbl[])  [unwired: 2 in, 2 out]
                n1805 = Number To Fractional String(number=w4489, width (-)=10, precision (6)=3) -> (F-format string=w4490:string[])  [unwired: 1 out]
              }
            }
            n1806 = case shown="False" w4471 {
              tunnel: w4480 -> [_ w4502]
              tunnel: [w4494 w4501] -> w4481
              tunnel: w4467 -> [_ w4500]
              tunnel: w4470 -> [_ w4499]
              tunnel: w4469 -> [_ w4498]
              frame False {
                w4496 = dbl[] [] ("Array 12")
                n1807 = Bundle("Array 12"=w4496, "Array 12"=w4496) -> (w4495:cluster{"Array 12":dbl[], "Array 12":dbl[]})  [unwired: 1 out]
                n1808 = Build Array(w4495) -> (w4494:cluster{"Array 12":dbl[], "Array 12":dbl[]}[])
              }
              frame True {
                n1809 = for {
                  tunnel: [w4511] -> w4501 mode=indexing
                  tunnel: w4502 -> [w4508]
                  tunnel: w4500 -> [_] mode=indexing
                  tunnel: w4499 -> [w4505]
                  tunnel: w4498 -> [w4504]
                  tunnel: w4498 -> [w4503]
                  i -> [w4509]
                  n1810 = case shown="4" w4505 {
                    tunnel: w4509 -> [w4515 w4521 w4526 w4532 w4537]
                    tunnel: w4508 -> [w4514 w4520 w4525 w4531 w4536]
                    tunnel: [w4513 w4519 w4524 w4528 w4535] -> w4507
                    tunnel: w4503 -> [w4512 w4517 w4522 w4527 w4533]
                    frame 0, Default {
                      n1811 = call "readbinary.vi"(7:w4512, "base path"=w4514, "file index"=w4515, "data column"="timi") -> ("data"=w4513:ext[])  [unwired: 7 out]
                    }
                    frame 1 {
                      n1812 = call "readbinary.vi"(7:w4517, "base path"=w4520, "file index"=w4521, "data column"="bdti") -> ("data"=w4519:ext[])  [unwired: 7 out]
                    }
                    frame 2 {
                      n1813 = call "readbinary.vi"(7:w4522, "base path"=w4525, "file index"=w4526, "data column"="bcli") -> ("data"=w4524:ext[])  [unwired: 7 out]
                    }
                    frame 3 {
                      n1814 = call "readbinary.vi"(7:w4527, "base path"=w4531, "file index"=w4532, "data column"="bcli") -> ("data"=w4529:ext[])  [unwired: 7 out]
                      n1815 = Reciprocal(x=w4529) -> (1/x=w4528:ext[])
                    }
                    frame 4 {
                      n1816 = call "readbinary.vi"(7:w4533, "base path"=w4536, "file index"=w4537, "data column"="dati") -> ("data"=w4535:ext[])  [unwired: 7 out]
                    }
                  }
                  n1817 = case shown="4" "y axis" {
                    tunnel: w4509 -> [w4541 w4547 w4552 w4558 w4563]
                    tunnel: w4508 -> [w4540 w4546 w4551 w4557 w4562]
                    tunnel: [w4539 w4545 w4550 w4554 w4561] -> w4506
                    tunnel: w4504 -> [w4538 w4543 w4548 w4553 w4559]
                    frame 0, Default {
                      n1818 = call "readbinary.vi"(7:w4538, "base path"=w4540, "file index"=w4541, "data column"="timi") -> ("data"=w4539:ext[])  [unwired: 7 out]
                    }
                    frame 1 {
                      n1819 = call "readbinary.vi"(7:w4543, "base path"=w4546, "file index"=w4547, "data column"="bdti") -> ("data"=w4545:ext[])  [unwired: 7 out]
                    }
                    frame 2 {
                      n1820 = call "readbinary.vi"(7:w4548, "base path"=w4551, "file index"=w4552, "data column"="bcli") -> ("data"=w4550:ext[])  [unwired: 7 out]
                    }
                    frame 3 {
                      n1821 = call "readbinary.vi"(7:w4553, "base path"=w4557, "file index"=w4558, "data column"="bcli") -> ("data"=w4555:ext[])  [unwired: 7 out]
                      n1822 = Reciprocal(x=w4555) -> (1/x=w4554:ext[])
                    }
                    frame 4 {
                      n1823 = call "readbinary.vi"(7:w4559, "base path"=w4562, "file index"=w4563, "data column"="dati") -> ("data"=w4561:ext[])  [unwired: 7 out]
                    }
                  }
                  n1824 = Bundle("data"=w4507, "data"=w4506) -> (w4511:cluster{"data":ext[], "data":ext[]})  [unwired: 1 out]
                }
                n1825 = global write "status.vi" "String"("plotting interpolation") -> ()
              }
            }
            "?" <- w4481
            n1826 = while {
              stop <- w4492 stop-if-true
              n1827 = Not(x="?") -> (.not. x?=w4492:bool)
              n1828 = Wait (ms)(milliseconds to wait=1000) -> ()  [unwired: 1 out]
            }
            n1829 = control-ref of="?"() -> (w4463:refnum<vi>)
            n1830 = call "Neilsetplot.vi"("Set axes names"=w4466, "max # rows (-1:all)"=-1, "Plot names"=w4464, "XYGraph Refnum"=w4463) -> ()  [unwired: 6 in, 2 out]
          }
          frame #6 {
            n1831 = Build Path(base path=w4567, name or relative path="files3") -> (appended path=w4573:path)
            n1832 = Build Path(base path=w4567, name or relative path="paths3") -> (appended path=w4570:path)
            n1833 = call-poly <vilib>:"Read From Spreadsheet File.vi"("file path (dialog if empty)"=w4570) -> ("first row"=w4568:string[])  [unwired: 3 in, 7 out]
            n1834 = Build Array("timi", "bdti", "bcli", "dati") -> (w4576:string[])
            n1835 = call-poly <vilib>:"Read From Spreadsheet File.vi"("file path (dialog if empty)"=w4573) -> ("first row"=w4572:string[])  [unwired: 3 in, 7 out]
            n1836 = String To Path(string=w4568) -> (path=w4569:path[])
            n1837 = case shown="True" "?" {
              tunnel: w4572 -> [_ w4594]
              tunnel: w4569 -> [_ w4593]
              tunnel: w4576 -> [_ w4592]
              tunnel: w4567 -> [_ w4591]
              tunnel: "file format" -> [_ w4590]
              tunnel: "append name" -> [_ w4589]
              tunnel: w4567 -> [_ w4585]
              tunnel: w4566 -> [_ w4588]
              tunnel: w4565 -> [w4583 w4587]
              tunnel: [w4583 w4586] -> w4564
              frame False {
              }
              frame True {
                n1838 = for {
                  tunnel: w4594 -> [w4611] mode=indexing
                  tunnel: w4593 -> [w4609] mode=indexing
                  tunnel: w4589 -> [w4610]
                  tunnel: w4592 -> [w4607]
                  tunnel: w4591 -> [w4605]
                  tunnel: w4590 -> [w4602]
                  tunnel: w4588 -> [w4601]
                  shift-right: [w4599] -> w4586
                  shift-left: w4587 -> [w4597]
                  tunnel: w4585 -> [w4596]
                  i -> [w4606]
                  n1839 = call "filecount.vi"("Path"=w4596) -> ("file count string"=w4595:string)  [unwired: 10 out]
                  n1840 = Concatenate Strings("mega", w4595, w4611, w4610) -> (w4608:string)
                  n1841 = Build Path(base path=w4609, name or relative path=w4608) -> (appended path=w4598:path)
                  n1842 = Build Array (concatenate)(w4598, w4597) -> (w4599:path[])
                  n1843 = for {
                    tunnel: w4607 -> [w4623] mode=indexing
                    tunnel: w4606 -> [w4626]
                    tunnel: w4605 -> [w4625]
                    tunnel: [w4624] -> w4603 mode=indexing
                    tunnel: w4601 -> [w4622]
                    n1844 = call "readbinary.vi"(7:w4622, "base path"=w4625, "file index"=w4626, "data column"=w4623) -> ("data"=w4624:ext[])  [unwired: 7 out]
                  }
                  n1845 = stacked-sequence {
                    tunnel: "time\tdB/dt\tBfield\tdata\n" -> [_ w4617 _]
                    tunnel: w4598 -> [w4612 w4616 w4620]
                    tunnel: w4603 -> [_ _ w4621]
                    tunnel: w4602 -> [_ _ w4618]
                    frame #0 {
                      n1846 = call <vilib>:"Check if File or Folder Exists.vi"("path"=w4612) -> ("file or folder exists?"=w4613:bool)  [unwired: 1 in, 9 out]
                      n1847 = case shown="True" w4613 {
                        selector: w4613 -> [_ w4615]
                        tunnel: w4612 -> [_ w4614]
                        frame False {
                        }
                        frame True {
                          n1848 = Delete(path (use dialog)=w4614, entire hierarchy (F)=w4615) -> ()  [unwired: 1 in, 5 out]
                        }
                      }
                    }
                    frame #1 {
                      n1849 = Write to Text File(file (use dialog)=w4616, text=w4617) -> ()  [unwired: 1 in, 4 out]
                    }
                    frame #2 {
                      w4619 = TRUE
                      n1850 = call "Write To Spreadsheet File2.vi"("transpose? (no:F)"=w4619, "format (%d)"=w4618, "append to file? (new file:F)"=w4619, "2D data"=w4621, "file path (dialog if empty)"=w4620) -> ()  [unwired: 3 in, 1 out]
                    }
                  }
                }
                n1851 = global write "status.vi" "String"("saving interpolation") -> ()
              }
            }
          }
        }
      }
      frame #7 {
        # "transform frame"
        n1852 = Or(x="?", y=w4630) -> (x .or. y?=w4631:bool)
        n1853 = stacked-sequence {
          tunnel: w4631 -> [_ w4690 _ _]
          tunnel: w4640 -> [w4644 w4689 w4891 w4948]
          tunnel: w4639 -> [_ w4688 _ _]
          tunnel: "spectrum type" -> [_ w4687 _ _]
          tunnel: "padding" -> [_ w4686 _ _]
          tunnel: "truncate spectrum" -> [_ w4685 _ _]
          tunnel: w4635 -> [_ _ w4899 _]
          tunnel: w4634 -> [_ w4684 _ _]
          tunnel: w4633 -> [w4641 w4683 w4889 w4947]
          tunnel: w4632 -> [w4642 _ _ _]
          tunnel: w4629 -> [_ _ _ w4946]
          tunnel: [_ _ _ w4945] -> w4628
          frame #0 {
            n1854 = Build Array("freq", "ampl", "phas") -> (w4645:string[])
            n1855 = Build Path(base path=w4644, name or relative path="files3") -> (appended path=w4646:path)
            n1856 = call-poly <vilib>:"Read From Spreadsheet File.vi"("file path (dialog if empty)"=w4646) -> ("first row"=w4643:string[])  [unwired: 3 in, 7 out]
            n1857 = stacked-sequence {
              tunnel: w4645 -> [w4653 w4664]
              tunnel: w4644 -> [w4652 w4663]
              tunnel: w4643 -> [w4651 w4665]
              tunnel: w4642 -> [_ w4660]
              tunnel: w4641 -> [_ w4661]
              frame #0 {
                n1858 = for {
                  tunnel: w4653 -> [w4656]
                  tunnel: w4652 -> [w4655]
                  tunnel: w4651 -> [_] mode=indexing
                  i -> [w4654]
                  n1859 = for {
                    tunnel: w4656 -> [w4659] mode=indexing
                    tunnel: w4655 -> [w4658]
                    tunnel: w4654 -> [w4657]
                    n1860 = call "createemptybinary.vi"("base path"=w4658, "file index"=w4657, "data column"=w4659) -> ()  [unwired: 9 out]
                  }
                }
              }
              frame #1 {
                n1861 = Equal?(x=w4661, y=w4660) -> (x = y?=w4662:bool)
                n1862 = case shown="False" w4662 {
                  tunnel: w4665 -> [w4670 _]
                  tunnel: w4664 -> [w4669 _]
                  tunnel: w4663 -> [w4668 _]
                  tunnel: w4660 -> [w4667 _]
                  tunnel: w4661 -> [w4666 _]
                  frame False {
                    n1863 = for {
                      tunnel: w4670 -> [_] mode=indexing
                      tunnel: w4669 -> [w4675]
                      tunnel: w4668 -> [w4673]
                      tunnel: w4667 -> [w4672]
                      tunnel: w4666 -> [w4671]
                      i -> [w4674]
                      n1864 = for {
                        tunnel: w4675 -> [w4678] mode=indexing
                        tunnel: w4674 -> [w4677]
                        tunnel: w4673 -> [w4676]
                        tunnel: w4672 -> [w4681]
                        tunnel: w4671 -> [w4679]
                        n1865 = call "readbinary.vi"(7:w4681, "base path"=w4676, "file index"=w4677, "data column"=w4678) -> ("data"=w4680:ext[])  [unwired: 7 out]
                        n1866 = call "writebinary.vi"(7:w4679, "base path"=w4676, "file index"=w4677, "data column"=w4678, "data"=w4680) -> ()  [unwired: 7 out]
                      }
                    }
                  }
                  frame True {
                  }
                }
              }
            }
          }
          frame #1 {
            n1867 = case shown="True" w4690 {
              tunnel: w4689 -> [_ w4698]
              tunnel: w4688 -> [_ w4697]
              tunnel: w4687 -> [_ w4696]
              tunnel: w4686 -> [_ w4695]
              tunnel: w4685 -> [_ w4694]
              tunnel: w4684 -> [_ w4693]
              tunnel: w4683 -> [_ w4692]
              tunnel: "Numeric" -> [_ w4691]
              frame False {
              }
              frame True {
                n1868 = stacked-sequence {
                  seq-local: [w4705 _ _] -> [_ w4724 w4852]
                  seq-local: [w4700 _ _] -> [_ w4721 _]
                  tunnel: w4698 -> [w4701 w4723 w4851]
                  tunnel: w4697 -> [_ w4722 _]
                  tunnel: w4696 -> [_ w4720 _]
                  tunnel: w4695 -> [_ w4719 _]
                  tunnel: w4694 -> [_ w4718 _]
                  tunnel: w4693 -> [_ w4717 _]
                  tunnel: w4692 -> [_ w4716 w4850]
                  tunnel: w4691 -> [_ w4715 _]
                  frame #0 {
                    n1869 = call "readbinary.vi"("base path"=w4701, "file index"=0, "data column"="inte") -> ("data"=w4703:ext[])  [unwired: 1 in, 7 out]
                    n1870 = Index Array(array=w4703) -> (element=w4700:ext)  [unwired: 1 in]
                    "interpolate in:" <- w4700
                    n1871 = Build Path(base path=w4701, name or relative path="paths3") -> (appended path=w4711:path)
                    n1872 = Build Path(base path=w4701, name or relative path="files3") -> (appended path=w4712:path)
                    n1873 = call-poly <vilib>:"Read From Spreadsheet File.vi"("file path (dialog if empty)"=w4711) -> ("first row"=w4706:string[])  [unwired: 3 in, 7 out]
                    n1874 = call-poly <vilib>:"Read From Spreadsheet File.vi"("file path (dialog if empty)"=w4712) -> ("first row"=w4705:string[])  [unwired: 3 in, 7 out]
                    n1875 = Build Path(base path=w4701, name or relative path="files4") -> (appended path=w4708:path)
                    n1876 = Build Path(base path=w4701, name or relative path="paths4") -> (appended path=w4707:path)
                    n1877 = global write "status.vi" "String"("transforming") -> ()
                    n1878 = call-poly <vilib>:"Write To Spreadsheet File.vi"("1D data"=w4705, "file path (dialog if empty)"=w4708) -> ()  [unwired: 4 in, 3 out]
                    n1879 = call-poly <vilib>:"Write To Spreadsheet File.vi"("1D data"=w4706, "file path (dialog if empty)"=w4707) -> ()  [unwired: 4 in, 3 out]
                  }
                  frame #1 {
                    n1880 = for {
                      tunnel: w4724 -> [_] mode=indexing
                      tunnel: w4723 -> [w4732]
                      tunnel: w4722 -> [w4737]
                      tunnel: w4721 -> [w4736]
                      tunnel: w4720 -> [w4735]
                      tunnel: w4719 -> [w4733]
                      tunnel: w4718 -> [w4731]
                      tunnel: w4717 -> [w4729]
                      tunnel: w4716 -> [w4728]
                      tunnel: w4715 -> [w4725]
                      i -> [w4730]
                      n1881 = case shown="1" w4737 {
                        tunnel: w4730 -> [w4832 w4837 w4843 w4848]
                        tunnel: w4732 -> [w4831 w4836 w4842 w4847]
                        tunnel: [w4830 w4835 w4840 w4846] -> w4734
